vi "ExCloseCamGlobal.vi"() -> ()   [LabVIEW 2010]
uses:
  GlbCamHndls.vi
panel:
  out "error out":errorcluster
  in  "error in (no error)":errorcluster
  # "ExCloseCamGlobal.vi : this sub vi closes the cameras for\nthe gloabal variable example."
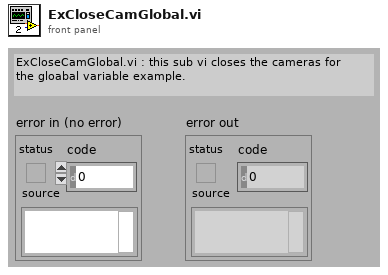
[diagram p1: front panel]
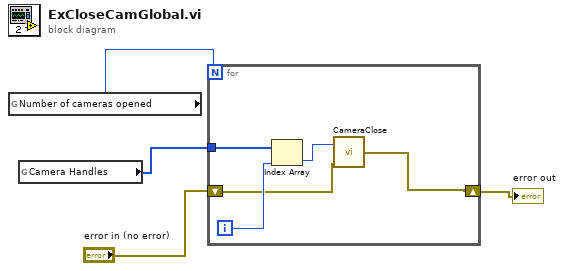
[diagram p0: block diagram]
diagram:
  n1 = global read "GlbCamHndls.vi" "Number of cameras opened"() -> (w4:u32)
  n2 = global read "GlbCamHndls.vi" "Camera Handles"() -> (w3:u32[])
  n3 = for {
    N: w4 -> [_]
    tunnel: w3 -> [w9]
    shift-right: [w5] -> w1
    shift-left: "error in (no error)" -> [w6]
    i -> [w8]
    n4 = Index Array(array=w9, index=w8) -> (element=w7:u32)
    n5 = call <userlib>:"CameraClose.vi"("error in"=w6, "Camera Handle"=w7) -> ("error out"=w5:errorcluster)
  }
  "error out" <- w1
